vi "9230ModulePresent.vi"(11 "all dynamic modules":string[](array[string])) -> (3 "9230 present":bool)   [LabVIEW 2017, in "CmsFpgaBitfileManager.lvlib"]
uses:
  <vilib>/addons/InsightCM/Devices/Shared/Cms/CmsFpgaBitfileManager/CmsFpgaBitfileManager.lvlib
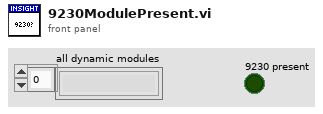
[diagram p1: front panel]
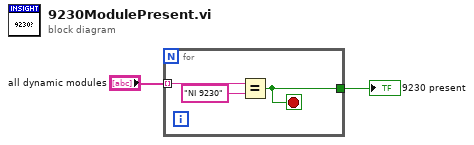
[diagram p0: block diagram]
diagram:
  n1 = for {
    tunnel: "all dynamic modules" -> [w5] mode=indexing
    tunnel: [w3] -> w1
    stop <- w3 stop-if-true
    n2 = Equal?(x=w5, y="NI 9230") -> (x = y?=w3:bool)
  }
  "9230 present" <- w1
